vi "openFile.vi"(0 "reference in":refnum<class "excelFile.lvclass">, 5 "error in (no error)":errorcluster) -> (14 "reference out":refnum<class "excelFile.lvclass">, 19 "error out":errorcluster)   [LabVIEW 2015, in "excelFile.lvclass"]
uses:
  excelFile.lvclass
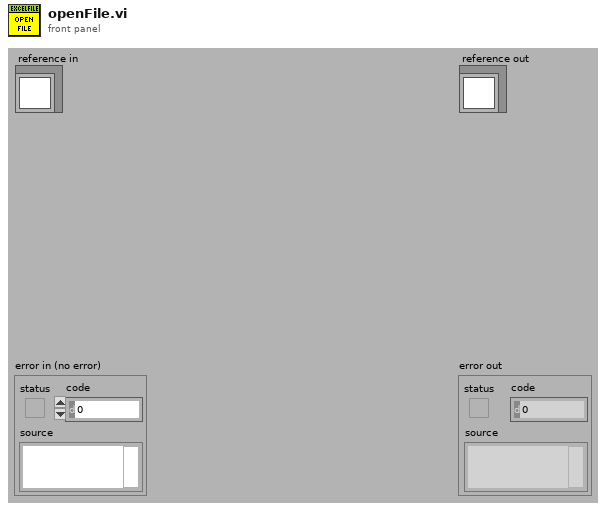
[diagram p1: front panel]
types:
  T1 = typedef "excelFile.lvclass/ObjectAttributesRef.ctl" = refnum<data-value>
  T2 = typedef "excelFile.lvclass/ObjectAttributes.ctl" = cluster{"MyAttribute":dbl, "path":string, "Refnum Excel":cluster{"Excel._Application":refnum<k7>, "Workbooks":refnum<k7>, "Open":refnum<k7>}, "data":string[][][], "save":bool, "fileType":T3, "rowsColor":u32[], "python_ref":refnum<class "python.lvclass">, "items_rows":i32[], "excel_range":i32[][], "TSR":cluster{"number":string, "TSR_path":path, "service_path":path}}
  T3 = typedef "excelFile.lvclass/fileType.ctl" = enum16{"devices", "items", "partsTracking", "TSR"}
  T4 = cluster{"Excel._Application":refnum<k7>, "Workbooks":refnum<k7>}
  T5 = cluster{"Excel._Application":refnum<k7>, "Workbooks":refnum<k7>, "Open":refnum<k7>}
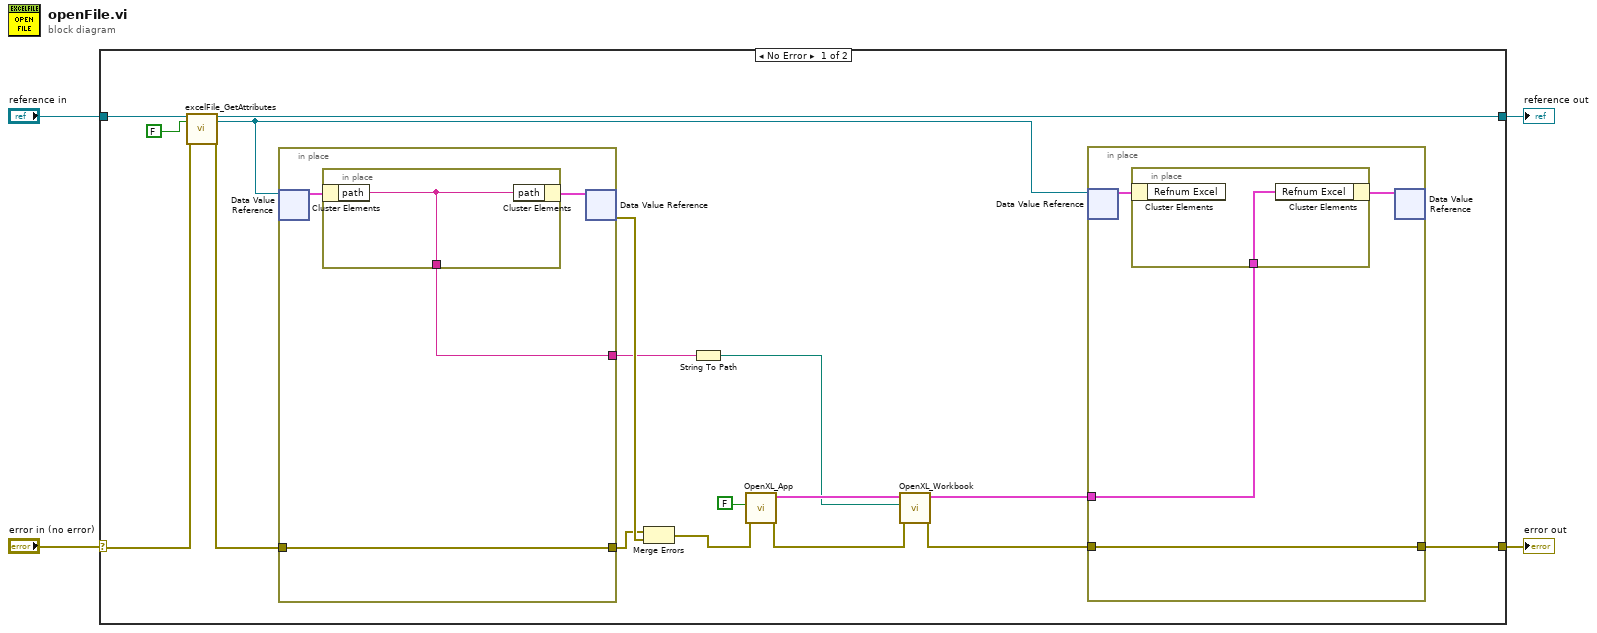
[diagram p0: block diagram]
diagram:
  n1 = case shown="No Error" "error in (no error)" {
    selector: "error in (no error)" -> [w17 w33]
    tunnel: [w13 w33] -> w3
    tunnel: [w15 w32] -> w1
    tunnel: "reference in" -> [w19 w32]
    frame No Error {
      n2 = call "excelFile_GetAttributes.vi"("reference in"=w19, "return data? (T)"=FALSE, "error in (no error)"=w17) -> ("reference out"=w15:refnum<class "excelFile.lvclass">, "attributes ref"=w12:T1, "error out"=w16:errorcluster)  [unwired: 13 in, 1 out]
      n3 = in-place {
        in-place-border: w16 -> [w28]
        in-place-border: [w28] -> w20
        in-place-border: [w27] -> w14
        n4 = in-place-dvr #1(w12) -> (w29:T2)  [unwired: 1 out]
        n5 = in-place {
          in-place-border: [w31] -> w27
          n6 = in-place-cluster #2(w29) -> ("path"=w31:string)
          n7 = in-place-cluster #2("path"=w31) -> (w30:T2)
        }
        n8 = in-place-dvr #1(w30) -> (w21:errorcluster)  [unwired: 1 out]
      }
      n9 = Merge Errors(w20, w21) -> (w11:errorcluster)
      n10 = String To Path(string=w14) -> (path=w7:path)
      n11 = call <userlib>:"OpenXL_App.vi"("error in (no error)"=w11, "Visible"=FALSE) -> ("error out"=w10:errorcluster, "Refnum Cluster"=w8:T4)  [unwired: 8 in]
      n12 = call <userlib>:"OpenXL_Workbook.vi"("error in"=w10, "path"=w7, "Refnum Cluster In"=w8) -> ("error out"=w9:errorcluster, "Refnum Cluster Out"=w6:T5)  [unwired: 7 in]
      n13 = in-place {
        in-place-border: w9 -> [w23]
        in-place-border: [w23] -> w13
        in-place-border: w6 -> [w22]
        n14 = in-place-dvr #3(w12) -> (w24:T2)  [unwired: 1 out]
        n15 = in-place {
          in-place-border: w22 -> [w26]
          n16 = in-place-cluster #4(w24) -> ()  [unwired: 1 out]
          n17 = in-place-cluster #4("Refnum Excel"=w26) -> (w25:T2)
        }
        n18 = in-place-dvr #3(w25) -> ()  [unwired: 2 out]
      }
    }
    frame Error {
    }
  }
  "error out" <- w3
  "reference out" <- w1
